vi "ModbusCRCCalculator.vi"(11 "ModbusCRCSettings":T1={"DataFIFO"="MockHPILCCRCDataFIFO", "CalculateFIFO"="MockHPILCCRCCalculateFIFO", "OutputFIFO"="MockHPILCCRCFIFO"}) -> ()   [LabVIEW 2016, in "FPGAModbus.lvlib"]
uses:
  FPGAModbus.lvlib
  DataTypes/ModbusCRCSettings.ctl
  <vilib>/rvi/Emulation/niFpgaGetClockAttributes.vi
  <vilib>/rvi/Emulation/niFpgaSctlEmulationGetInTimedLoop.vi
  <vilib>/rvi/Emulation/niFpgaEmulationReportErrorSimple.vi
  <vilib>/rvi/DataTransferAndStorage/Container/Common/niFpgaContainerExecOnDevCompGetState.vi
  <vilib>/rvi/Emulation/niFpgaEmulationIsFPGAContextNoSignature.vi
  <vilib>/rvi/errors/niFpgaSetErrorForExecOnDevCompSimple.vi
  <vilib>/rvi/eio/common/nirviEmuReportErrorAndStop.vi
  <vilib>/rvi/DataTransferAndStorage/Container/Common/niFpgaContainerGetUniqueNameForEmu.vi
  <vilib>/rvi/FIFO/Fifo_Resource/nirvififoEmulationSetSize.vi
  <vilib>/rvi/FIFO/Fifo_Resource/nirviFifoEmulationQueueMgr.vi
  <instcachedir>/0/nirviFifoEmulationQueueMgr_E5CAEC123FF24DC58D834DCA3CDAA9B5.lvgen/nirviFifoEmulationQueueMgr_E5CAEC123FF24DC58D834DCA3CDAA9B5_009.vi
  <vilib>/rvi/FIFO/Fifo_Resource/nirvififoEmulationDetermineInputValidOut.vi
  <vilib>/rvi/FIFO/Fifo_Resource/nirvififoEmulationCreateLock.vi
  <vilib>/rvi/Emulation/niFpgaProcessEmulError.vi
  <vilib>/rvi/FIFO/Fifo_Resource/nirvififoEmulationObtainLock.vi
  <vilib>/rvi/FIFO/Fifo_Resource/nirvififoEmulationReleaseLock.vi
  <vilib>/rvi/occurrence/nirviWaitOnOccurrenceBase.vi
  <vilib>/rvi/errors/nirviReportUnexpectedCaseInternalError.vi
  <vilib>/rvi/errors/nirviReportUnexpectedCaseInternalError (U32).vi
  <vilib>/Utility/error.llb/Clear Errors.vi
  <vilib>/rvi/interface/RandomDataEmulation/niFpgaRandomDataHandleErrors.vi
  <instcachedir>/0/nirviFifoEmulationQueueMgr_E5CAEC123FF24DC58D834DCA3CDAA9B5.lvgen/nirviFifoEmulationQueueMgr_E5CAEC123FF24DC58D834DCA3CDAA9B5_004.vi
  <vilib>/rvi/Emulation/niFpgaCriticalErrorInLSC.vi
  <vilib>/rvi/DataTransferAndStorage/Container/XNode/niFpgaContainer.xnode
  <vilib>/rvi/FIFO/Fifo_Resource/niFpgaFifoEmulationRefIn.vi
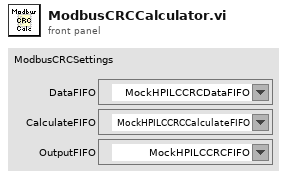
[diagram p1: front panel]
types:
  T1 = typedef "FPGAModbus.lvlib/ModbusCRCSettings.ctl" = cluster{"DataFIFO":refnum<k21>, "CalculateFIFO":refnum<k21>, "OutputFIFO":refnum<k21>}
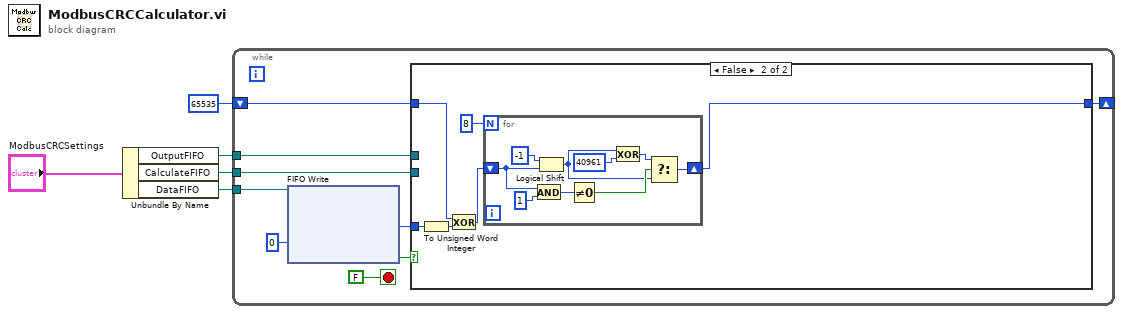
[diagram p0: block diagram]
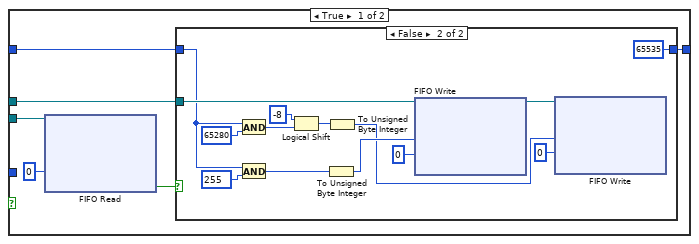
[diagram p2: hidden frame]
diagram:
  n1 = Unbundle By Name("ModbusCRCSettings") -> ("OutputFIFO"=w1:refnum<k21>, "CalculateFIFO"=w2:refnum<k21>, "DataFIFO"=w3:refnum<k21>)
  n2 = while {
    shift-right: [w8] -> _
    shift-left: u16 65535 -> [w11]
    tunnel: w3 -> [w14]
    tunnel: w2 -> [w9]
    tunnel: w1 -> [w7]
    stop <- FALSE stop-if-true
    n3 = xnode "FIFO Write"("Timeout"=0, "FIFO In"=w14) -> ("Element"=w12:u8, "Timed Out?"=w10:bool)  [unwired: 1 out]
    n4 = case shown="False" w10 {
      tunnel: w12 -> [_ w41]
      tunnel: w11 -> [w17 w39]
      tunnel: w9 -> [w20 _]
      tunnel: [w16 w36] -> w8
      tunnel: w7 -> [w15 _]
      frame True {
        n5 = xnode "FIFO Read"("Timeout"=0, "FIFO In"=w20) -> ("Timed Out?"=w18:bool)  [unwired: 2 out]
        n6 = case shown="False" w18 {
          tunnel: w17 -> [w21 w27]
          tunnel: [w21 u16 65535] -> w16
          tunnel: w15 -> [_ w35]
          frame True {
          }
          frame False {
            n7 = And(x=w27, y=u16 65280) -> (x .and. y?=w30:u16)
            n8 = And(x=w27, y=u16 255) -> (x .and. y?=w31:u16)
            n9 = Logical Shift(y=i16 -8, x=w30) -> (x << y=w25:u16)
            n10 = To Unsigned Byte Integer(number=w31) -> (unsigned 8bit integer=w23:u8)
            n11 = To Unsigned Byte Integer(number=w25) -> (unsigned 8bit integer=w22:u8)
            n12 = xnode "FIFO Write"("Element"=w23, "Timeout"=0, "FIFO In"=w35) -> ("FIFO Out"=w32:refnum<k21>)  [unwired: 1 out]
            n13 = xnode "FIFO Write"("Element"=w22, "Timeout"=0, "FIFO In"=w32) -> ()  [unwired: 2 out]
          }
        }
      }
      frame False {
        n14 = To Unsigned Word Integer(number=w41) -> (unsigned 16bit integer=w40:u16)
        n15 = Exclusive Or(1:w40, 2:w39) -> (0:w38:u16)
        n16 = for {
          N: 8 -> [_]
          shift-right: [w42] -> w36
          shift-left: w38 -> [w43]
          n17 = And(x=w43, y=u16 1) -> (x .and. y?=w50:u16)
          n18 = Logical Shift(y=i16 -1, x=w43) -> (x << y=w44:u16)
          n19 = Not Equal To 0?(x=w50) -> (x != 0?=w49:bool)
          n20 = Exclusive Or(1:u16 40961 ("y"), 2:w44) -> (0:w45:u16)
          n21 = Select(t=w45, s=w49, f=w44) -> (s? t:f=w42:u16)
        }
      }
    }
  }
